vi "小信号配置.vi"(10 "电流通道":u16(ring) items=["正常.IA", "小信号.UB", "小信号.IB", "小信号.UC"], 11 "串口号":refnum<visa-resource-name>) -> (9 "应答":string)   [LabVIEW 2014]
panel:
  out "完整帧":u8[](array[numeric]) format="%.0x"
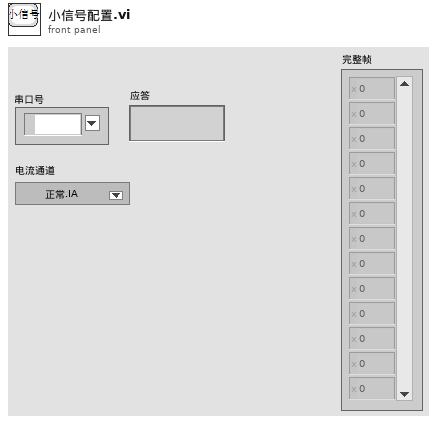
[diagram p1: front panel]
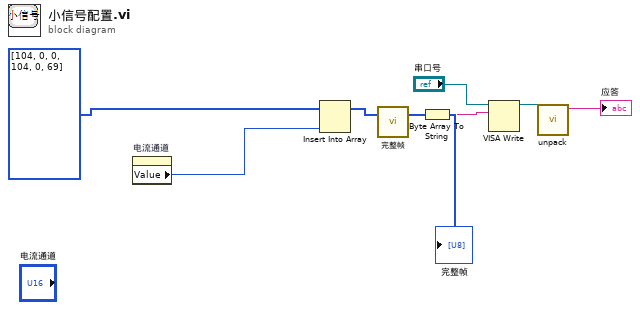
[diagram p0: block diagram]
diagram:
  n1 = property on="电流通道" class="Ring (严格)"() -> ("Value"=w1:u16)  [unwired: 2 in, 2 out]
  n2 = Insert Into Array(array=u8[] [104, 0, 0, 104, 0, 69], new element=w1) -> (w3:u8[])  [unwired: 1 in]
  n3 = call "完整帧.vi"("不完整帧"=w3) -> ("完整帧"=w8:u8[])  [unwired: 2 in]
  "完整帧" <- w8
  n4 = Byte Array To String(unsigned byte array=w8) -> (string=w7:string)
  n5 = VISA Write(VISA resource name="串口号", write buffer=w7) -> (VISA resource name out=w5:refnum<visa-resource-name>)  [unwired: 1 in, 2 out]
  n6 = call "unpack.vi"("串口号输入"=w5) -> ("应答"=→"应答":string)  [unwired: 5 in, 1 out]
